vi "Write State Sample Message.vi"(8 "error in (no error)":errorcluster, 10 "RDS State Tracker.lvlib:RDS State.lvclass":refnum<class "RDS State.lvclass">, 11 "State Sample Message in":refnum<class "State Sample Message.lvclass">) -> (0 "error out":errorcluster, 3 "State Sample Message out":refnum<class "State Sample Message.lvclass">)   [LabVIEW 2015, in "RDS Child Messages.lvlib" / "State Sample Message.lvclass"]
uses:
  State Sample Message.lvclass
  RDS State Tracker/RDS State/RDS State.lvclass
  State Sample Message.lvclass/State Sample Message.ctl
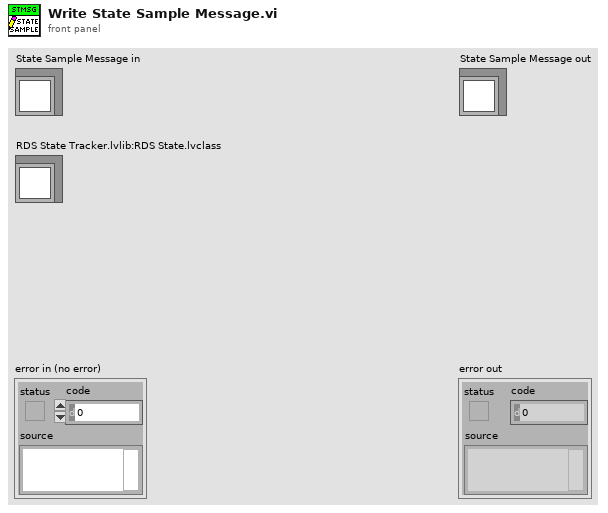
[diagram p1: front panel]
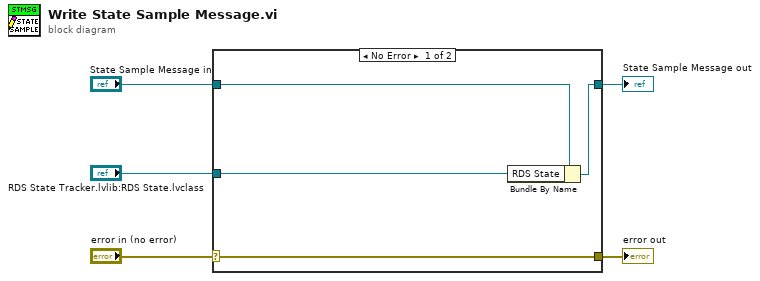
[diagram p0: block diagram]
diagram:
  n1 = case shown="No Error" "error in (no error)" {
    selector: "error in (no error)" -> [w9 w10]
    tunnel: [w9 w10] -> w4
    tunnel: [w7 w11] -> w2
    tunnel: "State Sample Message in" -> [w8 w11]
    tunnel: "RDS State Tracker.lvlib:RDS State.lvclass" -> [w6 _]
    frame No Error {
      n2 = Bundle By Name(cluster=w8, "RDS State"=w6) -> (w7:refnum<class "State Sample Message.lvclass">)
    }
    frame Error {
    }
  }
  "error out" <- w4
  "State Sample Message out" <- w2
